vi "GEA2_Reregister.vi"(5 "Board Index":i32 min=0 max=10 step=1, 7 "Event Registration In":refnum<event-registration>, 11 "Error In":errorcluster) -> (4 "GEA2 Reference Out":refnum<k24>, 6 "Board ID":string, 8 "Event Registration Out":refnum<event-registration>, 15 "Error Out":errorcluster)   [LabVIEW 2021]
uses:
  D:/Common/LabVIEW GEA2 Toolkit/source/GEA3 DLL Source/GeaCommunication.dll
  Common/LabVIEW GEA2 Toolkit/source/GEA3 DLL Source/GeaCommunication.dll
  Common/LabVIEW GEA2 Toolkit/GEA3/type defs/Data Out.ctl
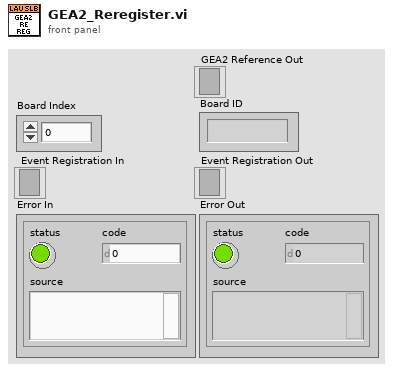
[diagram p1: front panel]
types:
  T1 = typedef "Data Out.ctl" = cluster{"Source":u8, "Destination":u8, "Command":u8, "Length":u8, "CRC":u16, "Message":string}
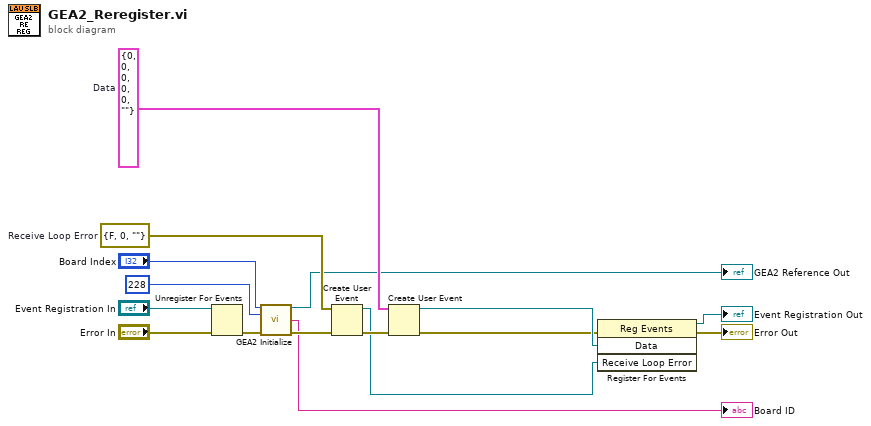
[diagram p0: block diagram]
diagram:
  w13 = errorcluster {"status"=FALSE, "code"=0, "source"=""}  # Receive Loop Error
  w14 = T1 {"Source"=0, "Destination"=0, "Command"=0, "Length"=0, "CRC"=0, "Message"=""}  # Data
  n1 = Unregister For Events(event registration refnum="Event Registration In", error in="Error In") -> (error out=w9:errorcluster)
  n2 = call "GEA2 Initialize.vi"("Board Index"="Board Index", "Source Address"=u8 228, "error in"=w9) -> ("GEA2 Reference Out"=→"GEA2 Reference Out":refnum<k24>, "Board ID"=→"Board ID":string, "error out"=w10:errorcluster)  [unwired: 10 in]
  n3 = Create User Event(user event datatype=w13, error in=w10) -> (user event=w11:refnum<user-event>, error out=w12:errorcluster)
  n4 = Create User Event(user event datatype=w14, error in=w12) -> (user event=w5:refnum<user-event>, error out=w1:errorcluster)
  n5 = register-events(error in=w1, w5, w11) -> (reference out=→"Event Registration Out":refnum<event-registration>, error out=→"Error Out":errorcluster)  [unwired: 1 in]
